vi "eeg.vi"(6 "channel_select_debug":string, 7 "LabVIEW Web Service Request":refnum<class "Web Request.lvclass">) -> (0 "eeg_stream_ch8":string, 1 "eeg_stream_ch7":string, 2 "eeg_stream_ch6":string, 3 "eeg_stream_ch5":string, 8 "eeg_stream_ch4":string, 9 "eeg_stream_ch3":string, 10 "eeg_stream_ch2":string, 11 "eeg_stream_ch1":string)   [LabVIEW 2020]
uses:
  <vilib>/wsapi/Web Request.lvclass
  Global 1.vi
panel:
  # "Use the Web Service Request input terminal to call the VIs on the Web Services palette. Do not remove it from the connector pane unless you don't need access to the palette."
  # "Each additional control wired to the connector pane will be available as an input in the URL. To include an indicator in terminal-mode output (the default setting), it must also be wired to the connector pane."
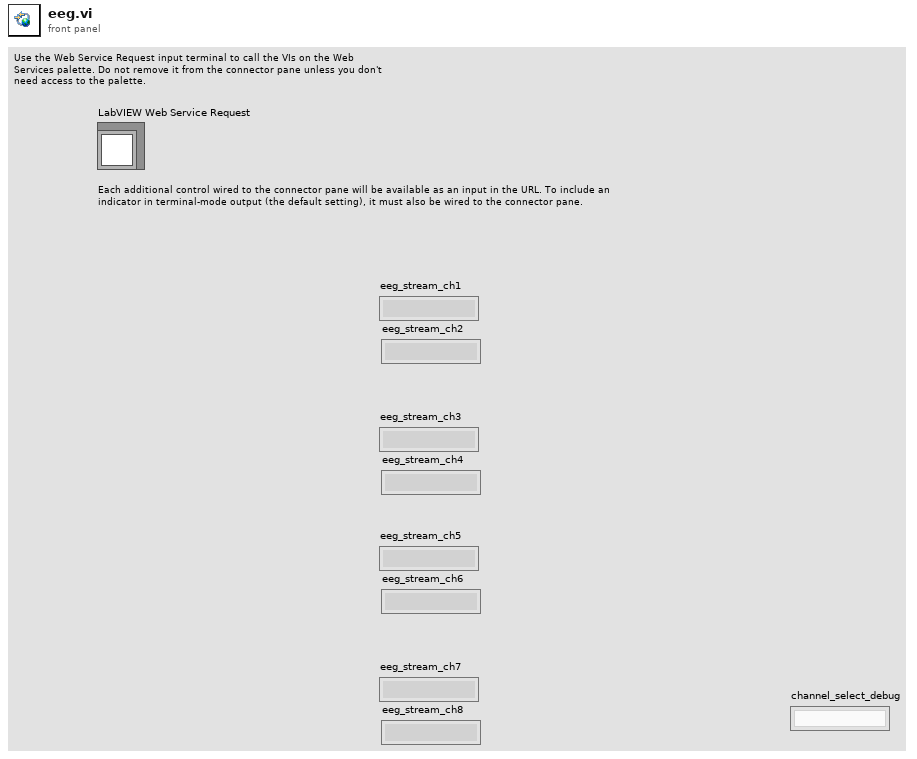
[diagram p1: front panel]
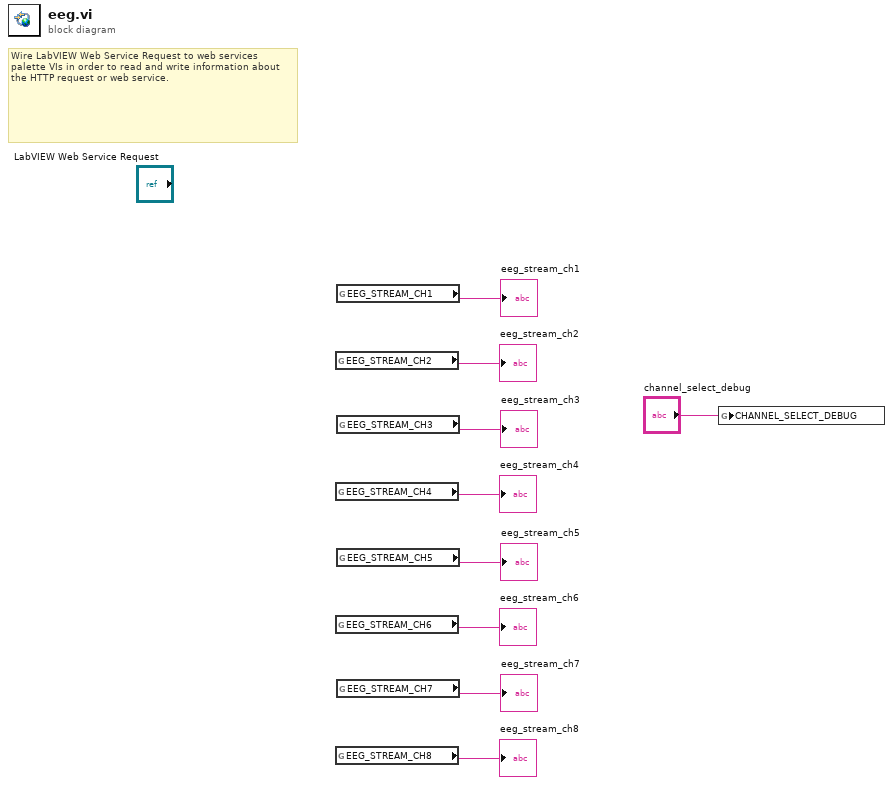
[diagram p0: block diagram]
diagram:
  # "Wire LabVIEW Web Service Request to web services palette VIs in order to read and write information about the HTTP request or web service."
  n1 = global read "Global 1.vi" "EEG_STREAM_CH2"() -> (→"eeg_stream_ch2":string)
  n2 = global read "Global 1.vi" "EEG_STREAM_CH4"() -> (→"eeg_stream_ch4":string)
  n3 = global read "Global 1.vi" "EEG_STREAM_CH6"() -> (→"eeg_stream_ch6":string)
  n4 = global read "Global 1.vi" "EEG_STREAM_CH8"() -> (→"eeg_stream_ch8":string)
  n5 = global read "Global 1.vi" "EEG_STREAM_CH1"() -> (→"eeg_stream_ch1":string)
  n6 = global read "Global 1.vi" "EEG_STREAM_CH3"() -> (→"eeg_stream_ch3":string)
  n7 = global read "Global 1.vi" "EEG_STREAM_CH5"() -> (→"eeg_stream_ch5":string)
  n8 = global read "Global 1.vi" "EEG_STREAM_CH7"() -> (→"eeg_stream_ch7":string)
  n9 = global write "Global 1.vi" "CHANNEL_SELECT_DEBUG"("channel_select_debug") -> ()
